vi "PLC_Simulation.vi"() -> ()   [LabVIEW 2017]
uses:
  Controls/PLC_DATA_READ.ctl
panel:
  in  "Stop":bool
  in  "Error Status in PLC Loop":errorcluster
  in  "PLC to Labview Data":i32[](array[numeric])
  in  "Send data":bool
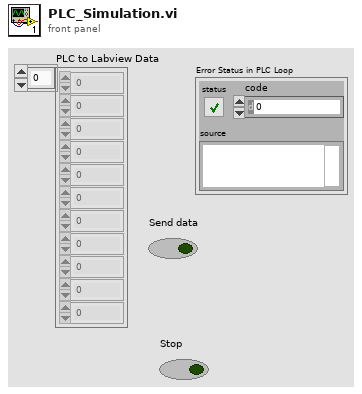
[diagram p1: front panel]
types:
  T1 = typedef "PLC_DATA_READ.ctl" = cluster{"PLC to Labview Data":i32[], "Error Status in PLC Loop":errorcluster}
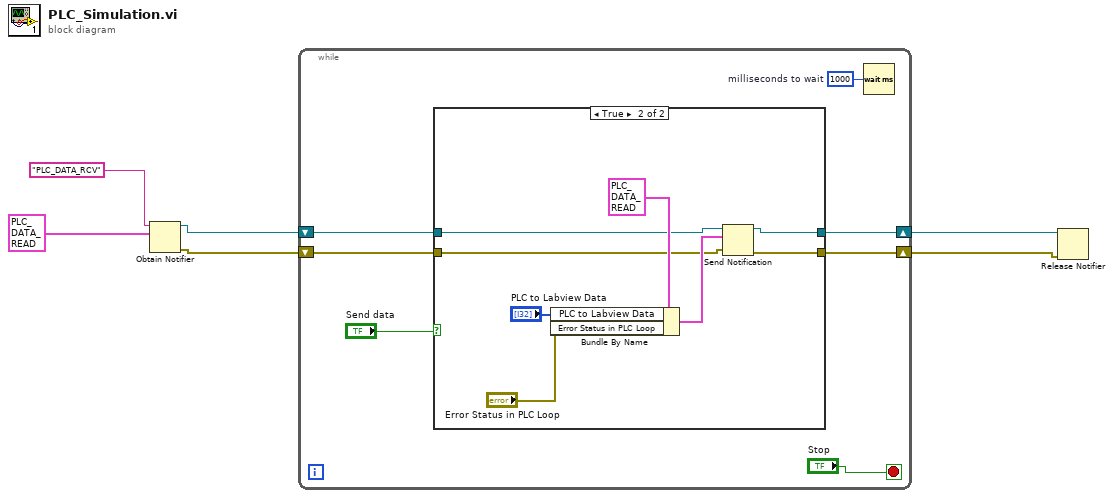
[diagram p0: block diagram]
diagram:
  n1 = Obtain Notifier(name (unnamed)="PLC_DATA_RCV", notification data type=T1 {"PLC to Labview Data"=[0, 0, 0, 0, 0, 0, 0, 0, 0, 0, 0, 0, 0, 0, 0], "Error Status in PLC Loop"={"status"=FALSE, "code"=0, "source"=""}}) -> (notifier out=w4:refnum<notifier>, error out=w1:errorcluster)  [unwired: 2 in, 1 out]
  n2 = while {
    shift-right: [w12] -> w3
    shift-left: w4 -> [w13]
    shift-right: [w11] -> w2
    shift-left: w1 -> [w10]
    stop <- "Stop" stop-if-true
    w9 = u32 1000  # milliseconds to wait
    n3 = case shown="True" "Send data" {
      tunnel: w13 -> [w14 w21]
      tunnel: [w14 w20] -> w12
      tunnel: [w15 w19] -> w11
      tunnel: w10 -> [w15 w18]
      frame False {
      }
      frame True {
        n4 = Bundle By Name(cluster=T1 {"PLC to Labview Data"=[0, 0, 0, 0, 0, 0, 0, 0, 0, 0, 0, 0, 0, 0, 0], "Error Status in PLC Loop"={"status"=FALSE, "code"=0, "source"=""}}, "PLC to Labview Data"="PLC to Labview Data", "Error Status in PLC Loop"="Error Status in PLC Loop") -> (w23:T1)
        n5 = Send Notification(notification=w23, notifier=w21, error in (no error)=w18) -> (notifier out=w20:refnum<notifier>, error out=w19:errorcluster)
      }
    }
    n6 = Wait (ms)(milliseconds to wait=w9) -> ()  [unwired: 1 out]
  }
  n7 = Release Notifier(notifier=w3, error in (no error)=w2) -> ()  [unwired: 1 in, 3 out]
